vi "Read Current (Linear Voltage Sweep).vi"(5 "Delay Time (0.01 S)":dbl=0.01, 6 "Pulse Stop Level (1 V)":dbl=1.0, 7 "Sweep Points (10)":i32=10, 8 "error in (no error)":errorcluster, 9 "Pulse Start Level (0 V)":dbl, 10 "Source Measure Unit Channel (0: Channel A)":i32(ring) items=["Channel A", "Channel B"], 11 "VISA resource name":refnum<visa-resource-name>) -> (0 "error out":errorcluster, 2 "Current (A)":dbl[](array[numeric]), 3 "VISA resource name out":refnum<visa-resource-name>)   [LabVIEW 2020, in "Keithley 2600 Series.lvlib"]
doc: "Performs a linear voltage sweep with current measured at every point."
uses:
  <instrlib>/Keithley 2600 Series/Keithley 2600 Series.lvlib
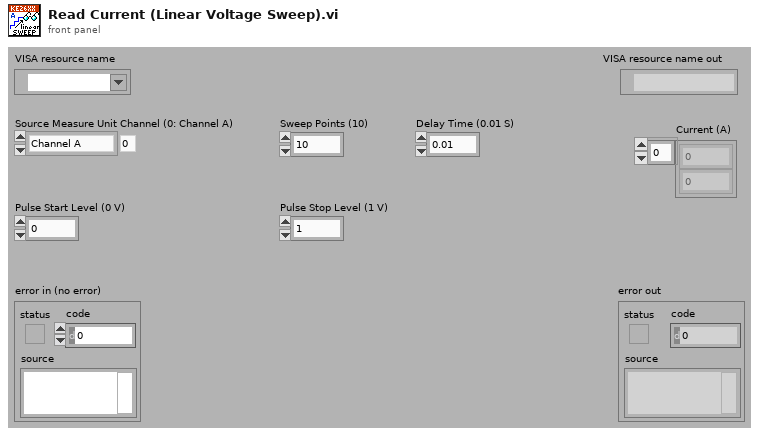
[diagram p1: front panel]
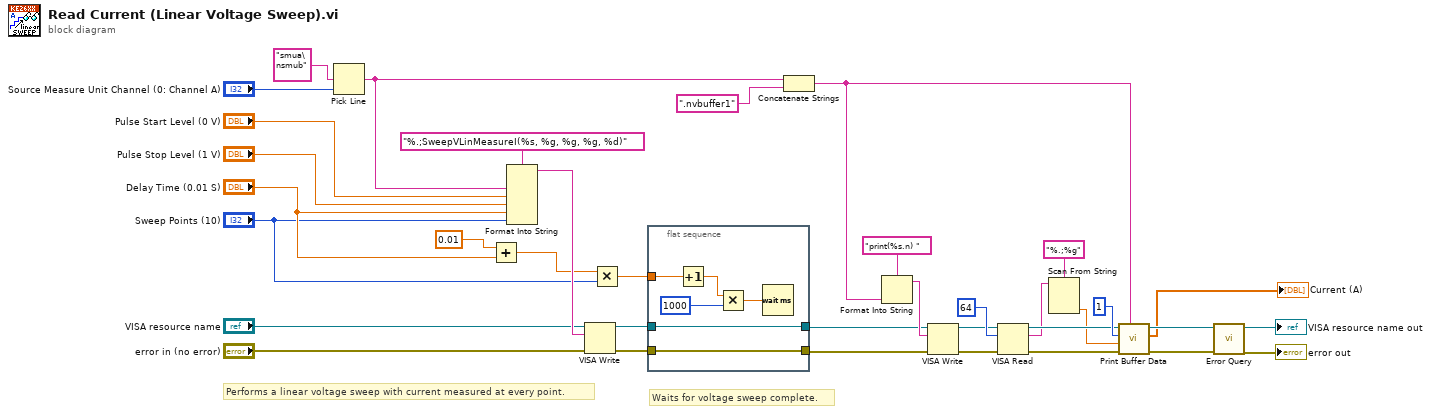
[diagram p0: block diagram]
diagram:
  # "Waits for voltage sweep complete."
  # "Performs a linear voltage sweep with current measured at every point."
  n1 = Pick Line(multi-line string="smua\nsmub", line index="Source Measure Unit Channel (0: Channel A)") -> (output string=w2:string)  [unwired: 1 in]
  n2 = Add(x=0.01, y="Delay Time (0.01 S)") -> (x+y=w21:dbl)
  n3 = Format Into String(format string="%.;SweepVLinMeasureI(%s, %g, %g, %g, %d)", w2, "Pulse Start Level (0 V)", "Pulse Stop Level (1 V)", "Delay Time (0.01 S)", "Sweep Points (10)") -> (resulting string=w33:string)  [unwired: 2 in, 1 out]
  n4 = VISA Write(VISA resource name="VISA resource name", write buffer=w33, error in (no error)="error in (no error)") -> (VISA resource name out=w26:refnum<visa-resource-name>, error out=w25:errorcluster)  [unwired: 1 out]
  n5 = Multiply(x=w21, y="Sweep Points (10)") -> (x*y=w24:dbl)
  n6 = flat-sequence {
    tunnel: w26 -> [w42]
    tunnel: w25 -> [w41]
    tunnel: [w42] -> w6
    tunnel: [w41] -> w5
    tunnel: w24 -> [w40]
    frame #0 {
      n7 = Increment(x=w40) -> (x+1=w37:dbl)
      n8 = Multiply(x=w37, y=1000) -> (x*y=w38:dbl)
      n9 = Wait (ms)(milliseconds to wait=w38) -> ()  [unwired: 1 out]
    }
  }
  n10 = Concatenate Strings(w2, ".nvbuffer1" ("string")) -> (w7:string)
  n11 = Format Into String(format string="print(%s.n) ", w7) -> (resulting string=w9:string)  [unwired: 2 in, 1 out]
  n12 = VISA Write(VISA resource name=w6, write buffer=w9, error in (no error)=w5) -> (VISA resource name out=w12:refnum<visa-resource-name>, error out=w11:errorcluster)  [unwired: 1 out]
  n13 = VISA Read(VISA resource name=w12, byte count=u32 64, error in (no error)=w11) -> (VISA resource name out=w17:refnum<visa-resource-name>, read buffer=w15:string, error out=w16:errorcluster)  [unwired: 1 out]
  n14 = Scan From String(format string="%.;%g", input string=w15) -> (output 1=w14:dbl)  [unwired: 3 in, 3 out]
  n15 = call <instrlib>:"Print Buffer Data.vi"("Reading Buffer (smua.nvbuffer1)"=w7, "error in (no error)"=w16, "End Index (1)"=w14, "Start Index (1)"=1 ("Start Index (0)"), "VISA resource name"=w17) -> ("error out"=w4:errorcluster, "Buffer Data"=→"Current (A)":dbl[], "VISA resource name out"=w3:refnum<visa-resource-name>)  [unwired: 4 in]
  n16 = call <instrlib>:"Error Query.vi"("error in (no error)"=w4, "VISA resource name"=w3) -> ("error out"=→"error out":errorcluster, "VISA resource name out"=→"VISA resource name out":refnum<visa-resource-name>)  [unwired: 6 in, 2 out]
